vi "moveBkt (SubVI).vi"(11 "Bkt stroke(mm)":sgl) -> (3 "bkt angle(deg)":sgl)   [LabVIEW 2020]
uses:
  <vilib>/imath/engines/lvmath2/RunTimeEngine/BuiltInFunctions/cos/NIMS_cos(C).vi
  <instcachedir>/0/NIMS_cos(C)_9DC0D0878EF24EB8B280F2BED1FF8FCD.lvgen/NIMS_cos(C)_9DC0D0878EF24EB8B280F2BED1FF8FCD_001.vi
  <vilib>/imath/engines/lvmath2/RunTimeEngine/ArithmeticOperatorToken/NIMS_ArithmeticOperator_power(S).vi
  <instcachedir>/0/NIMS_ArithmeticOperator_power(S)_0FB4C2FA3CD746849DC4699515FAC284.lvgen/NIMS_ArithmeticOperator_power(S)_0FB4C2FA3CD746849DC4699515FAC284_010.vi
  <vilib>/imath/engines/lvmath2/RunTimeEngine/BuiltInFunctions/acos/NIMS_acos(C).vi
  <instcachedir>/0/NIMS_acos(C)_5BB0E87CCFB0408A9DC8B350AC83525E.lvgen/NIMS_acos(C)_5BB0E87CCFB0408A9DC8B350AC83525E_001.vi
  <vilib>/imath/engines/lvmath2/RunTimeEngine/ErrorHandling/NIMS_Create Error From Enums.vi
  <vilib>/imath/engines/lvmath2/RunTimeEngine/NodeEndStatement/NIMS_NodeEndStatement_Output.vi
  <instcachedir>/0/NIMS_NodeEndStatement_Output_53EC0D466D134D7ABD903AC30B43404B.lvgen/NIMS_NodeEndStatement_Output_53EC0D466D134D7ABD903AC30B43404B_009.vi
  <vilib>/imath/engines/lvmath2/RunTimeEngine/ErrorHandling/NIMS_Finalize Error.vi
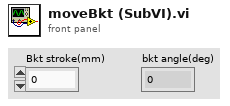
[diagram p1: front panel]
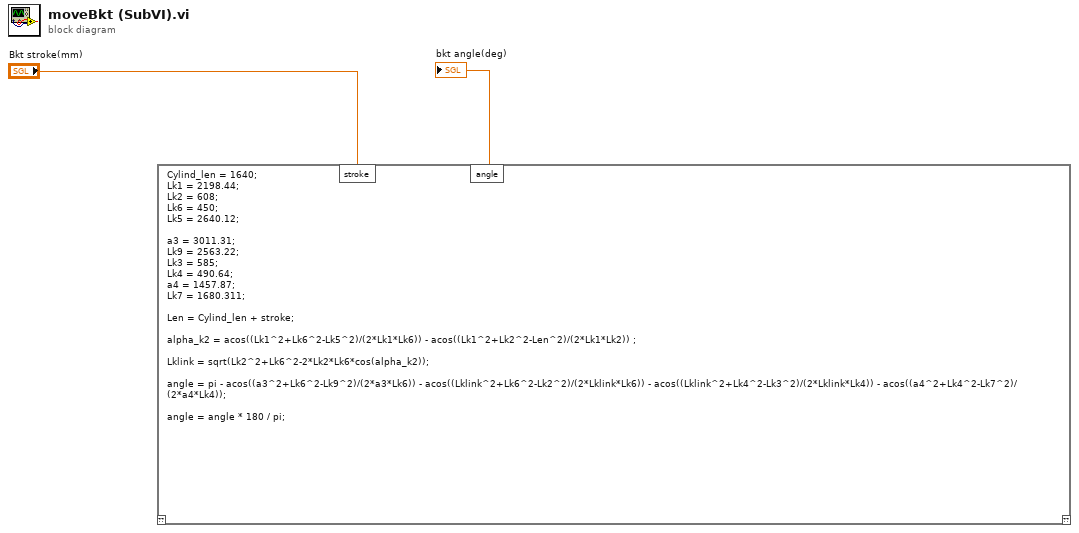
[diagram p0: block diagram]
diagram:
  n1 = mathscript code="Cylind_len = 1640;\nLk1 = 2198.44;\nLk2 = 608;\nLk6 = 450;\nLk5 = 2640.12;\n\na3 = 3011.31;\nLk9 = 2563.22;\nLk3 = 585;\nLk4 = 490.64;\na4 = 1457.87;\nLk7 = 1680.311;\n\nLen = Cylind_len + stroke;\n\nalpha_k2 = acos((Lk1^2+Lk6^2-Lk5^2)/(2*Lk1*Lk6)) - acos((Lk1^2+Lk2^2-Len^2)/(2*Lk1*Lk2)) ;\n\nLklink = sqrt(Lk2^2+Lk6^2-2*Lk2*Lk6*cos(alpha_k2));\n\nangle = pi - acos((a3^2+Lk6^2-Lk9^2)/(2*a3*Lk6)) - acos((Lklink^2+Lk6^2-Lk2^2)/(2*Lklink*Lk6)) - acos((Lklink^2+Lk4^2-Lk3^2)/(2*Lklink*Lk4)) - acos((a4^2+Lk4^2-Lk7^2)/(2*a4*Lk4));\n\nangle = angle * 180 / pi;"("stroke"="Bkt stroke(mm)") -> ("angle"=→"bkt angle(deg)":cdb)  [unwired: 1 in, 1 out]
